vi "Barcode_Write_DTU.vi"(7 "queue IN":refnum<queue>, 8 "error in (no error)":errorcluster, 10 "CAN_Frames.CAN_ID":u32, 11 "Barcode":string="ADDGSC000001") -> (0 "error out":errorcluster)   [LabVIEW 2024, in "Test_2.lvlib"]
uses:
  Test_2.lvlib
  PCANusb_DTU/support/CAN_MSGs.ctl
  PCANusb_DTU/support/CAN_Frames_ctrl.ctl
  PCANusb_DTU/support/Framing datas.ctl
  PCANusb_DTU/PCANusb_DTU.lvlib
panel:
  out "Barcode_Send":u8[][](array[numeric]) format="%.0x"
  out "unsigned byte array":u8[](array[numeric]) format="%.0x"
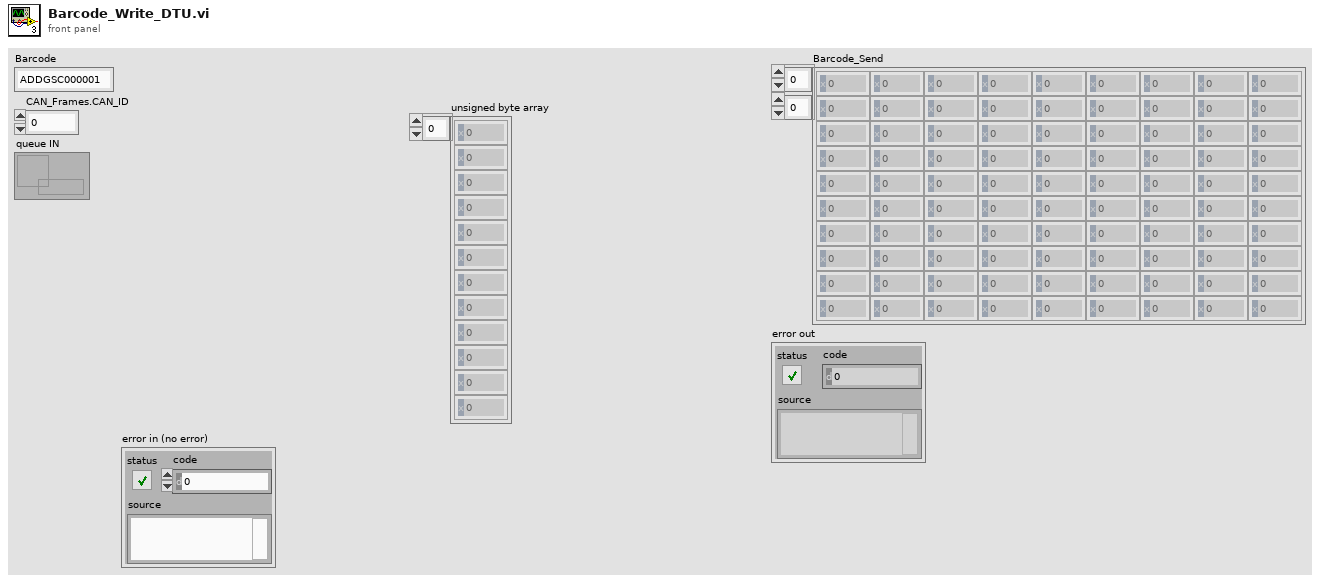
[diagram p1: front panel]
types:
  T1 = typedef "PCANusb_DTU.lvlib/CAN_MSGs.ctl" = cluster{"Scaling Factor":u16, "Physical value":dbl, "CAN_Frames":T2, "Offset value":dbl, "Framing datas":T3[], "CAN_Frame Enable":bool, "Add Signal":bool, "Delete Signal":bool, "Signal Values":dbl[], "Time(ms)":dbl, "Repetition":bool, "Delay":bool, "Delay time":dbl}
  T2 = typedef "PCANusb_DTU.lvlib/CAN_Frames_ctrl.ctl" = cluster{"CAN_ID":u32, "MSGTYPE":u8, "Payload":u8[], "Length":u8}
  T3 = typedef "PCANusb_DTU.lvlib/Framing datas.ctl" = cluster{"Signal name":string, "Start Bit":u8, "Length":u8, "Value":u16}
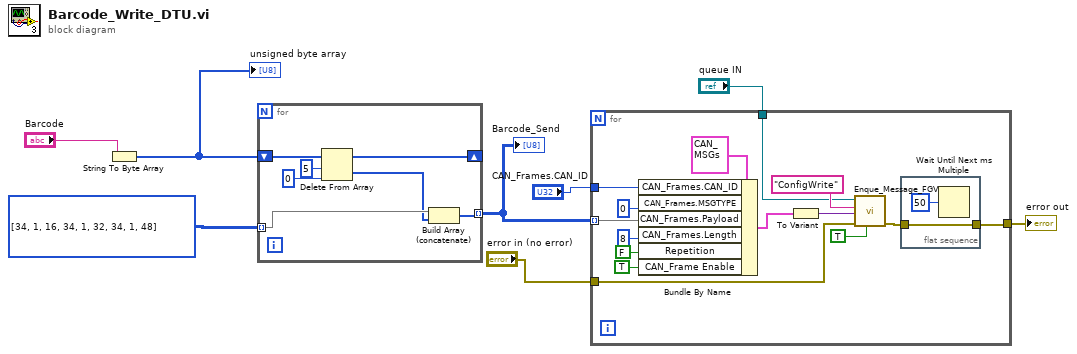
[diagram p0: block diagram]
diagram:
  n1 = String To Byte Array(string="Barcode") -> (unsigned byte array=w6:u8[])
  "unsigned byte array" <- w6
  n2 = for {
    tunnel: u8[][] [[34, 1, 16], [34, 1, 32], [34, 1, 48]] -> [w11] mode=indexing
    shift-right: [w12] -> _
    shift-left: w6 -> [w15]
    tunnel: [w9] -> w5 mode=indexing
    n3 = Delete From Array(array=w15, length=5, index=0) -> (deleted portion=w10:u8[], array with subset deleted=w12:u8[])
    n4 = Build Array (concatenate)(w11, w10) -> (w9:u8[])
  }
  "Barcode_Send" <- w5
  n5 = for {
    tunnel: w5 -> [w21] mode=indexing
    tunnel: "CAN_Frames.CAN_ID" -> [w20]
    tunnel: [w17] -> w2
    tunnel: "error in (no error)" -> [w19]
    tunnel: "queue IN" -> [w16]
    n6 = Bundle By Name(cluster=T1 {"Scaling Factor"=1, "Physical value"=0.0, "CAN_Frames"={"CAN_ID"=0, "MSGTYPE"=128, "Payload"=[], "Length"=0}, "Offset value"=0.0, "Framing datas"=[], "CAN_Frame Enable"=FALSE, "Add Signal"=FALSE, "Delete Signal"=FALSE, "Signal Values"=[], "Time(ms)"=0.0, "Repetition"=FALSE, "Delay"=FALSE, "Delay time"=0.0} ("CAN_MSGs"), "CAN_Frames.CAN_ID"=w20, "CAN_Frames.MSGTYPE"=u8 0, "CAN_Frames.Payload"=w21, "CAN_Frames.Length"=u8 8, "Repetition"=FALSE, "CAN_Frame Enable"=TRUE) -> (w25:T1)
    n7 = To Variant(anything=w25) -> (Variant=w24:variant)
    n8 = call "Enque_Message_FGV.vi"("Priority"=TRUE, "error in (no error)"=w19, "Message Data"=w24, "Message"="ConfigWrite", "queue IN"=w16) -> ("error out"=w18:errorcluster)  [unwired: 6 in]
    n9 = flat-sequence {
      tunnel: w18 -> [w31]
      tunnel: [w31] -> w17
      frame #0 {
        n10 = Wait Until Next ms Multiple(millisecond multiple=u32 50) -> ()  [unwired: 1 out]
      }
    }
  }
  "error out" <- w2
